vi "LEDs state machine 123.vi"() -> ()   [LabVIEW 2013]
panel:
  out "Three":bool
  in  "NumberValue":dbl
  out "Two":bool
  out "One":bool
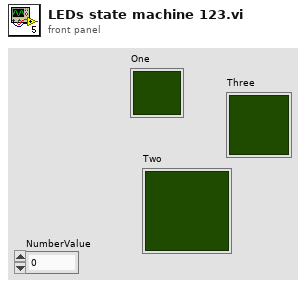
[diagram p1: front panel]
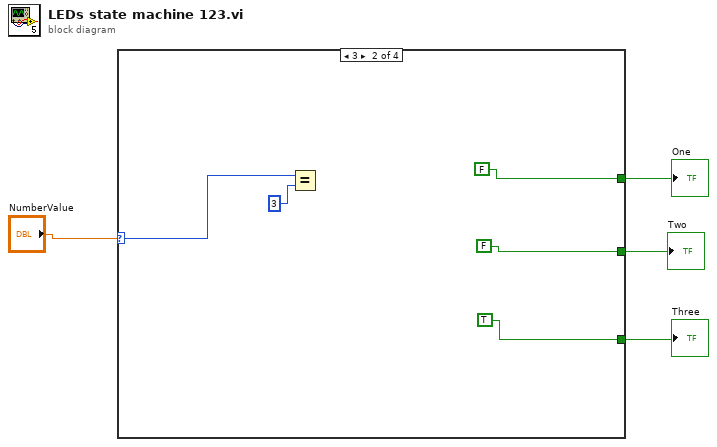
[diagram p0: block diagram]
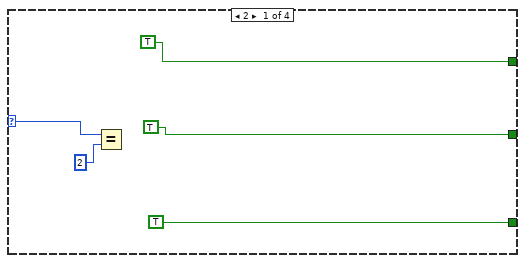
[diagram p2: hidden frame]
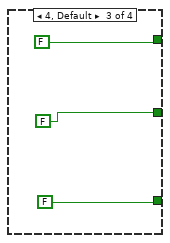
[diagram p3: hidden frame]
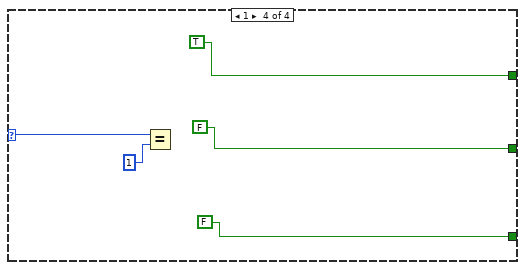
[diagram p4: hidden frame]
diagram:
  n1 = case shown="3" "NumberValue" {
    selector: "NumberValue" -> [w9 w13 _ w21]
    tunnel: [TRUE FALSE FALSE TRUE] -> w1
    tunnel: [TRUE FALSE FALSE FALSE] -> w3
    tunnel: [TRUE TRUE FALSE FALSE] -> w2
    frame 2 {
      n2 = Equal?(x=w9, y=2) -> ()  [unwired: 1 out]
    }
    frame 3 {
      n3 = Equal?(x=w13, y=3) -> ()  [unwired: 1 out]
    }
    frame 4, Default {
    }
    frame 1 {
      n4 = Equal?(x=w21, y=1) -> ()  [unwired: 1 out]
    }
  }
  "Three" <- w2
  "Two" <- w3
  "One" <- w1
